vi "Radians to Pot Volts.vi"(1 "Angle In":dbl) -> (0 "Pot Delta Out":dbl)   [LabVIEW 2012]
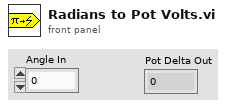
[diagram p1: front panel]
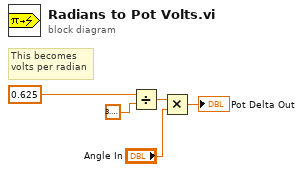
[diagram p0: block diagram]
diagram:
  # "This becomes\nvolts per radian"
  n1 = Divide(x=0.625, y=3.141592653589793) -> (x/y=w4:dbl)
  n2 = Multiply(x=w4, y="Angle In") -> (x*y=→"Pot Delta Out":dbl)
